vi "V_ShapeDetectResultTable.vi"(8 "error in (no error)":errorcluster, 10 "Result":variant, 11 "Shape Type":T2(ring)) -> (0 "error out":errorcluster, 2 "Result":T1)   [LabVIEW 2019]
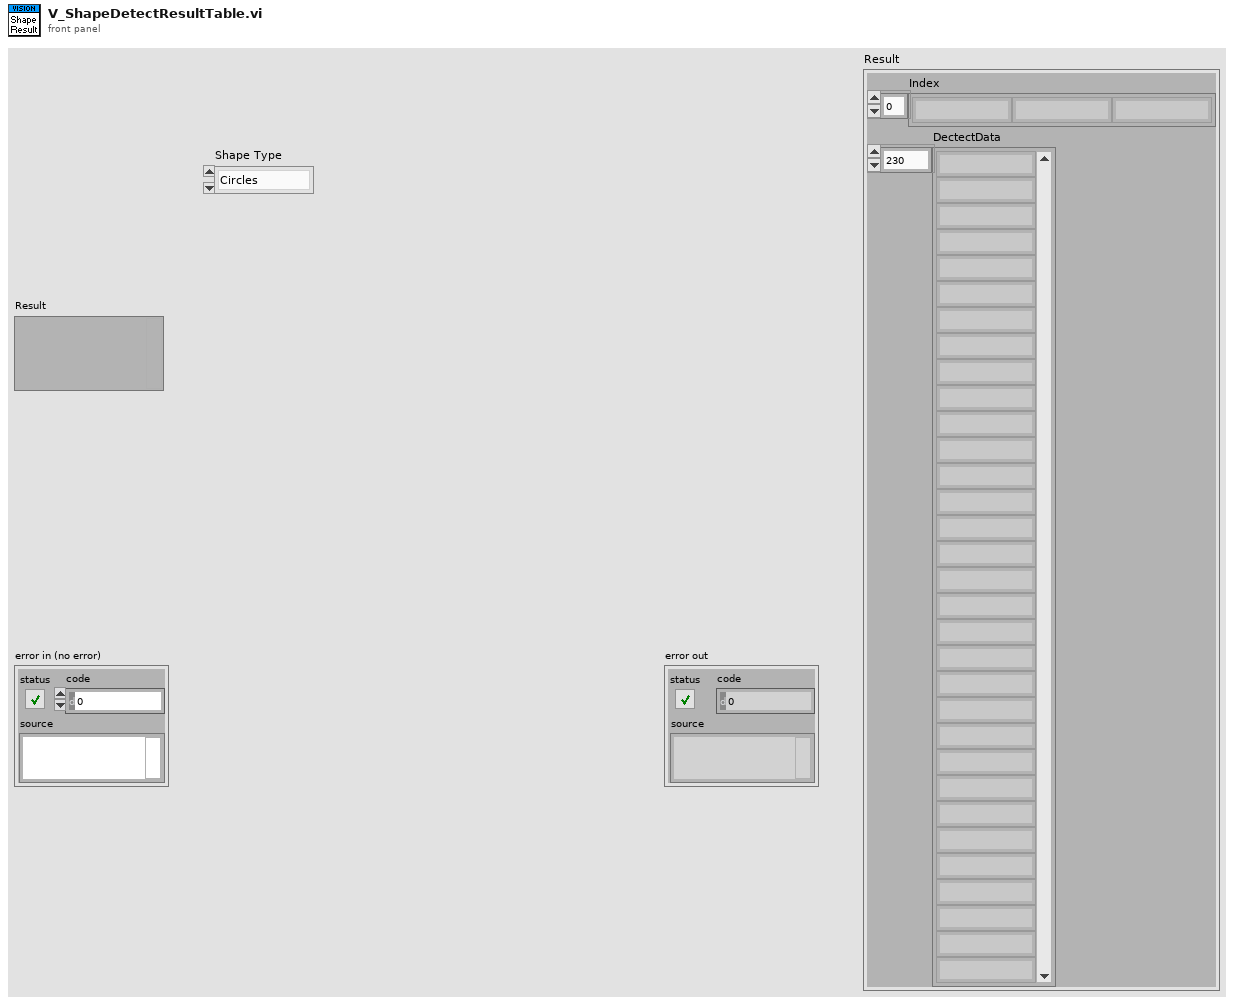
[diagram p1: front panel]
types:
  T1 = cluster{"Index":string[], "DectectData":string[]}
  T2 = enum16{"Circles", "Ellipses", "Lines", "Rectangles"}
  T3 = cluster{"Position":cluster{"X":sgl, "Y":sgl}, "Radius":dbl, "Score":dbl}[]
  T4 = cluster{"Circles":cluster{"Position":cluster{"X":sgl, "Y":sgl}, "Radius":dbl, "Score":dbl}[], "Circles (Calibrated)":cluster{"Position":cluster{"X":sgl, "Y":sgl}, "Radius":dbl, "Score":dbl}[]}
  T5 = cluster{"Pixel":cluster{"Position":cluster{"X":sgl, "Y":sgl}, "Angle":dbl, "Major Radius":dbl, "Minor Radius":dbl, "Score":dbl}[], "Ellipses (Calibrated)":cluster{"Position":cluster{"X":sgl, "Y":sgl}, "Orientation":dbl, "Major Radius":dbl, "Minor Radius":dbl, "Score":dbl}[]}
  T6 = cluster{"Position":cluster{"X":sgl, "Y":sgl}, "Angle":dbl, "Major Radius":dbl, "Minor Radius":dbl, "Score":dbl}[]
  T7 = cluster{"Position":cluster{"X":sgl, "Y":sgl}, "Orientation":dbl, "Major Radius":dbl, "Minor Radius":dbl, "Score":dbl}[]
  T8 = cluster{"Lines":cluster{"Start Point":cluster{"X":sgl, "Y":sgl}, "End Point":cluster{"X":sgl, "Y":sgl}, "Length":dbl, "Angle":dbl, "Score":dbl}[], "Lines Calibrated":cluster{"Start Point":cluster{"X":sgl, "Y":sgl}, "End Point":cluster{"X":sgl, "Y":sgl}, "Length":dbl, "Orientation":dbl, "Score":dbl}[]}
  T9 = cluster{"Start Point":cluster{"X":sgl, "Y":sgl}, "End Point":cluster{"X":sgl, "Y":sgl}, "Length":dbl, "Angle":dbl, "Score":dbl}[]
  T10 = cluster{"Start Point":cluster{"X":sgl, "Y":sgl}, "End Point":cluster{"X":sgl, "Y":sgl}, "Length":dbl, "Orientation":dbl, "Score":dbl}[]
  T11 = cluster{"Rectangles":cluster{"Corners":cluster{"X":sgl, "Y":sgl}[], "Angle":dbl, "Width":dbl, "Height":dbl, "Score":dbl}[], "Rectangles Calibrated":cluster{"Corners":cluster{"X":sgl, "Y":sgl}[], "Angle":dbl, "Width":dbl, "Height":dbl, "Score":dbl}[]}
  T12 = cluster{"Corners":cluster{"X":sgl, "Y":sgl}[], "Angle":dbl, "Width":dbl, "Height":dbl, "Score":dbl}[]
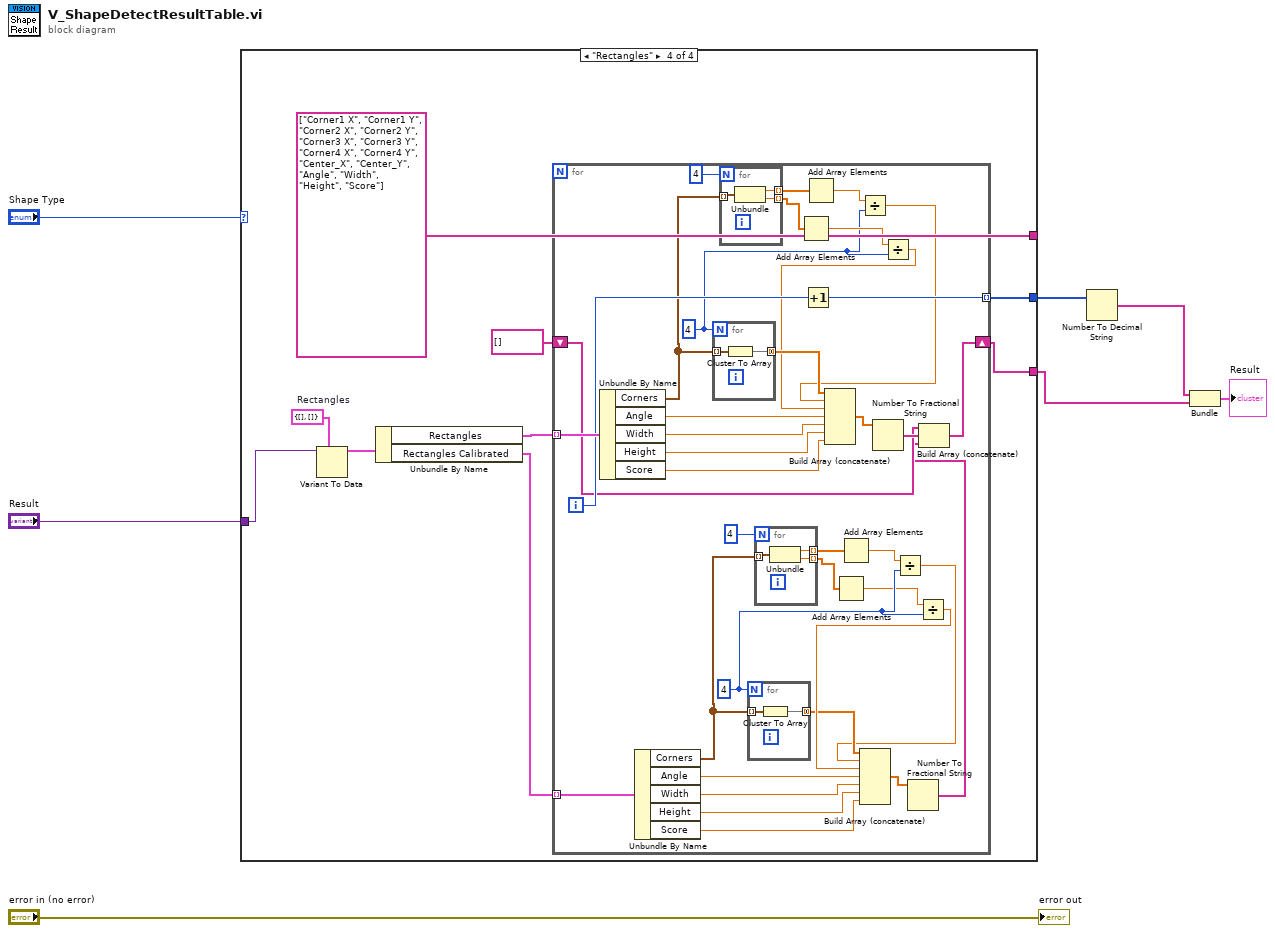
[diagram p0: block diagram]
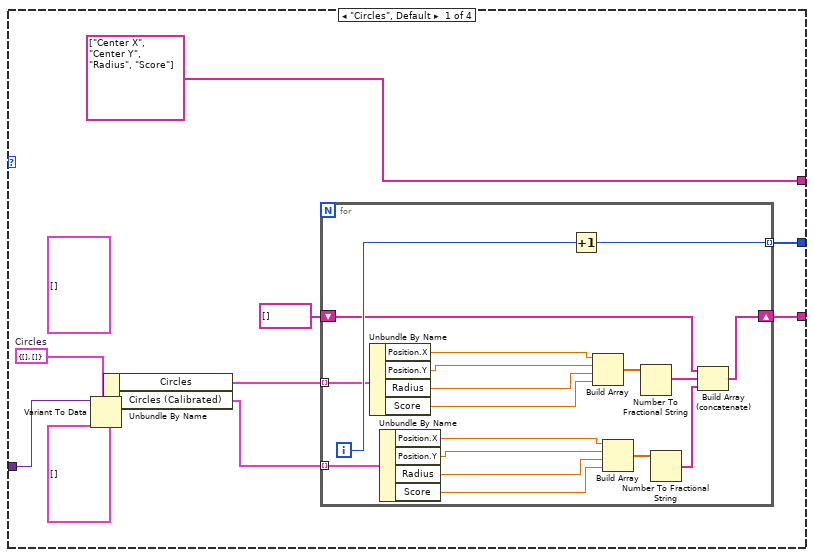
[diagram p2: hidden frame]
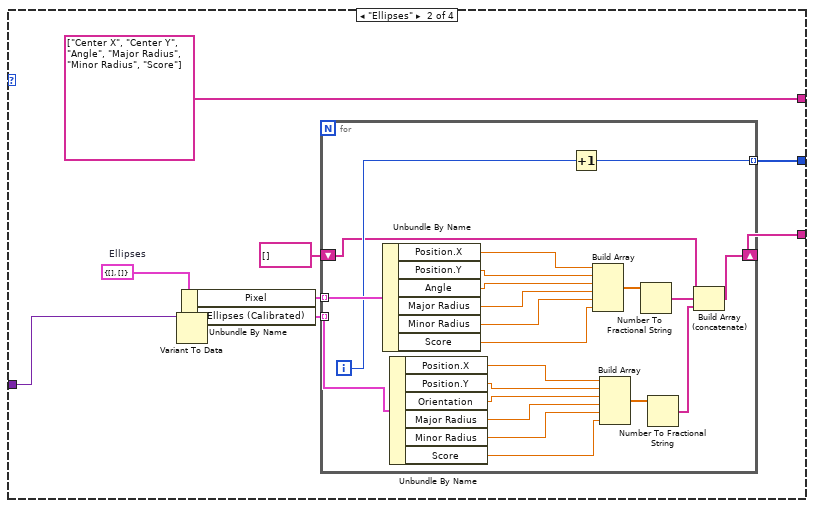
[diagram p3: hidden frame]
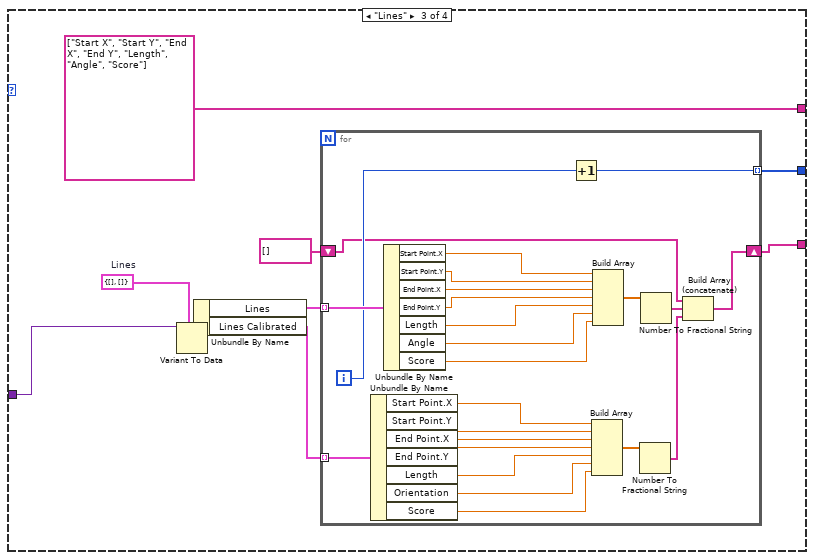
[diagram p4: hidden frame]
diagram:
  n1 = case shown="\"Rectangles\"" "Shape Type" {
    tunnel: [string[] ["Center X", "Center Y", "Radius", "Score"] string[] ["Center X", "Center Y", "Angle", "Major Radius", "Minor Radius", "Score"] string[] ["Start X", "Start Y", "End X", "End Y", "Length", "Angle", "Score"] string[] ["Corner1 X", "Corner1 Y", "Corner2 X", "Corner2 Y", "Corner3 X", "Corner3 Y", "Corner4 X", "Corner4 Y", "Center_X", "Center_Y", "Angle", "Width", "Height", "Score"]] -> _
    tunnel: "Result" -> [w15 w41 w73 w104]
    tunnel: [w12 w38 w69 w102] -> w4
    tunnel: [w10 w37 w68 w101] -> w1
    frame "Circles", Default {
      (unwired) T3 [] ("Circles (Calibrated)")
      (unwired) T3 [] ("Circles")
      w14 = T4 {"Circles"=[], "Circles (Calibrated)"=[]}  # Circles
      n2 = Variant To Data(type=w14, Variant=w15) -> (data=w13:T4)  [unwired: 1 in, 1 out]
      n3 = Unbundle By Name(w13) -> ("Circles"=w9:T3, "Circles (Calibrated)"=w8:T3)
      n4 = for {
        tunnel: [w29] -> w12 mode=indexing
        shift-right: [w25] -> w10
        shift-left: string[] [] -> [w26]
        tunnel: w9 -> [w24] mode=indexing
        tunnel: w8 -> [w19] mode=indexing
        i -> [w30]
        n5 = Unbundle By Name(w24) -> ("Position.X"=w28:sgl, "Position.Y"=w34:sgl, "Radius"=w32:dbl, "Score"=w33:dbl)
        n6 = Unbundle By Name(w19) -> ("Position.X"=w17:sgl, "Position.Y"=w20:sgl, "Radius"=w22:dbl, "Score"=w21:dbl)
        n7 = Increment(x=w30) -> (x+1=w29:i32)
        n8 = Build Array(w28, w34, w32, w33) -> (w31:dbl[])
        n9 = Build Array(w17, w20, w22, w21) -> (w23:dbl[])
        n10 = Number To Fractional String(number=w31) -> (F-format string=w27:string[])  [unwired: 3 in]
        n11 = Number To Fractional String(number=w23) -> (F-format string=w18:string[])  [unwired: 3 in]
        n12 = Build Array (concatenate)(w26, w27, w18) -> (w25:string[])
      }
    }
    frame "Ellipses" {
      w42 = T5 {"Pixel"=[], "Ellipses (Calibrated)"=[]}  # Ellipses
      n13 = Variant To Data(type=w42, Variant=w41) -> (data=w40:T5)  [unwired: 1 in, 1 out]
      n14 = Unbundle By Name(w40) -> ("Pixel"=w39:T6, "Ellipses (Calibrated)"=w35:T7)
      n15 = for {
        tunnel: w39 -> [w65] mode=indexing
        tunnel: [w59] -> w38 mode=indexing
        shift-right: [w54] -> w37
        shift-left: string[] [] -> [w53]
        tunnel: w35 -> [w45] mode=indexing
        i -> [w60]
        n16 = Unbundle By Name(w65) -> ("Position.X"=w58:sgl, "Position.Y"=w64:sgl, "Angle"=w63:dbl, "Major Radius"=w56:dbl, "Minor Radius"=w55:dbl, "Score"=w57:dbl)
        n17 = Unbundle By Name(w45) -> ("Position.X"=w46:sgl, "Position.Y"=w47:sgl, "Orientation"=w48:dbl, "Major Radius"=w51:dbl, "Minor Radius"=w52:dbl, "Score"=w50:dbl)
        n18 = Increment(x=w60) -> (x+1=w59:i32)
        n19 = Build Array(w58, w64, w63, w56, w55, w57) -> (w62:dbl[])
        n20 = Build Array(w46, w47, w48, w51, w52, w50) -> (w49:dbl[])
        n21 = Number To Fractional String(number=w62) -> (F-format string=w61:string[])  [unwired: 3 in]
        n22 = Number To Fractional String(number=w49) -> (F-format string=w44:string[])  [unwired: 3 in]
        n23 = Build Array (concatenate)(w53, w61, w44) -> (w54:string[])
      }
    }
    frame "Lines" {
      w72 = T8 {"Lines"=[], "Lines Calibrated"=[]}  # Lines
      n24 = Variant To Data(type=w72, Variant=w73) -> (data=w71:T8)  [unwired: 1 in, 1 out]
      n25 = Unbundle By Name(w71) -> ("Lines"=w70:T9, "Lines Calibrated"=w66:T10)
      n26 = for {
        tunnel: w70 -> [w98] mode=indexing
        tunnel: [w93] -> w69 mode=indexing
        shift-right: [w86] -> w68
        shift-left: string[] [] -> [w85]
        tunnel: w66 -> [w77] mode=indexing
        i -> [w94]
        n27 = Unbundle By Name(w77) -> ("Start Point.X"=w76:sgl, "Start Point.Y"=w78:sgl, "End Point.X"=w79:sgl, "End Point.Y"=w82:sgl, "Length"=w83:dbl, "Orientation"=w81:dbl, "Score"=w84:dbl)
        n28 = Unbundle By Name(w98) -> ("Start Point.X"=w89:sgl, "Start Point.Y"=w97:sgl, "End Point.X"=w96:sgl, "End Point.Y"=w91:sgl, "Length"=w90:dbl, "Angle"=w92:dbl, "Score"=w88:dbl)
        n29 = Increment(x=w94) -> (x+1=w93:i32)
        n30 = Build Array(w76, w78, w79, w82, w83, w81, w84) -> (w80:dbl[])
        n31 = Build Array(w89, w97, w96, w91, w90, w92, w88) -> (w95:dbl[])
        n32 = Number To Fractional String(number=w80) -> (F-format string=w75:string[])  [unwired: 3 in]
        n33 = Number To Fractional String(number=w95) -> (F-format string=w87:string[])  [unwired: 3 in]
        n34 = Build Array (concatenate)(w85, w87, w75) -> (w86:string[])
      }
    }
    frame "Rectangles" {
      w105 = T11 {"Rectangles"=[], "Rectangles Calibrated"=[]}  # Rectangles
      n35 = Variant To Data(type=w105, Variant=w104) -> (data=w103:T11)  [unwired: 1 in, 1 out]
      n36 = Unbundle By Name(w103) -> ("Rectangles"=w106:T12, "Rectangles Calibrated"=w99:T12)
      n37 = for {
        tunnel: w106 -> [w145] mode=indexing
        tunnel: [w137] -> w102 mode=indexing
        shift-right: [w136] -> w101
        shift-left: string[] [] -> [w135]
        tunnel: w99 -> [w110] mode=indexing
        i -> [w138]
        w122 = 4
        w128 = 4
        n38 = Unbundle By Name(w145) -> ("Corners"=w133:cluster{"X":sgl, "Y":sgl}[], "Angle"=w144:dbl, "Width"=w141:dbl, "Height"=w142:dbl, "Score"=w143:dbl)
        n39 = Unbundle By Name(w110) -> ("Corners"=w117:cluster{"X":sgl, "Y":sgl}[], "Angle"=w111:dbl, "Width"=w114:dbl, "Height"=w113:dbl, "Score"=w112:dbl)
        n40 = for {
          N: w128 -> [_]
          tunnel: w133 -> [w155] mode=indexing
          tunnel: [w154] -> w127 mode=concatenating
          n41 = Cluster To Array(cluster=w155) -> (array=w154:sgl[])
        }
        n42 = for {
          N: 4 -> [_]
          tunnel: w133 -> [w153] mode=indexing
          tunnel: [w152] -> w132 mode=indexing
          tunnel: [w151] -> w131 mode=indexing
          n43 = Unbundle(w153) -> ("X"=w152:sgl, "Y"=w151:sgl)
        }
        n44 = for {
          N: w122 -> [_]
          tunnel: w117 -> [w150] mode=indexing
          tunnel: [w149] -> w123 mode=concatenating
          n45 = Cluster To Array(cluster=w150) -> (array=w149:sgl[])
        }
        n46 = for {
          N: 4 -> [_]
          tunnel: w117 -> [w148] mode=indexing
          tunnel: [w147] -> w118 mode=indexing
          tunnel: [w146] -> w119 mode=indexing
          n47 = Unbundle(w148) -> ("X"=w147:sgl, "Y"=w146:sgl)
        }
        n48 = Add Array Elements(numeric array=w131) -> (sum=w129:sgl)
        n49 = Increment(x=w138) -> (x+1=w137:i32)
        n50 = Add Array Elements(numeric array=w132) -> (sum=w130:sgl)
        n51 = Add Array Elements(numeric array=w119) -> (sum=w121:sgl)
        n52 = Add Array Elements(numeric array=w118) -> (sum=w120:sgl)
        n53 = Divide(x=w130, y=w128) -> (x/y=w126:sgl)
        n54 = Divide(x=w129, y=w128) -> (x/y=w125:sgl)
        n55 = Build Array (concatenate)(w127, w126, w125, w144, w141, w142, w143) -> (w140:dbl[])
        n56 = Number To Fractional String(number=w140) -> (F-format string=w139:string[])  [unwired: 3 in]
        n57 = Divide(x=w120, y=w122) -> (x/y=w109:sgl)
        n58 = Divide(x=w121, y=w122) -> (x/y=w124:sgl)
        n59 = Build Array (concatenate)(w123, w109, w124, w111, w114, w113, w112) -> (w115:dbl[])
        n60 = Number To Fractional String(number=w115) -> (F-format string=w108:string[])  [unwired: 3 in]
        n61 = Build Array (concatenate)(w135, w139, w108) -> (w136:string[])
      }
    }
  }
  n62 = Number To Decimal String(number=w4) -> (decimal integer string=w3:string[])  [unwired: 1 in]
  n63 = Bundle(w3, w1) -> (→"Result":cluster{string[], string[]})  [unwired: 1 in]
  "error out" <- "error in (no error)"
